vi "Get Names.vi"(11 "Stock":T1[](array[typedef])) -> (2 "Product Names":string[](array[string]))   [LabVIEW 2019, in "Stock.lvlib"]
uses:
  Stock.lvlib
  Products.ctl
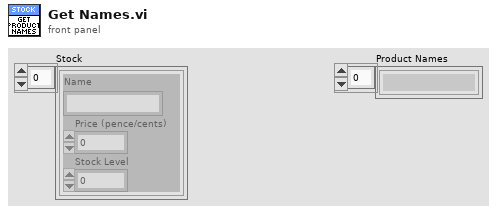
[diagram p1: front panel]
types:
  T1 = typedef "Stock.lvlib/Products.ctl" = cluster{"Name":string, "Price (pence/cents)":u32, "Stock Level":u32}
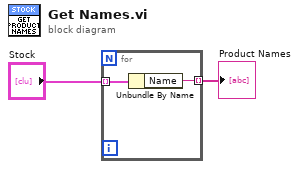
[diagram p0: block diagram]
diagram:
  n1 = for {
    tunnel: "Stock" -> [w4] mode=indexing
    tunnel: [w3] -> w2 mode=indexing
    n2 = Unbundle By Name(w4) -> ("Name"=w3:string)
  }
  "Product Names" <- w2
